vi "Initialize.vi"(8 "error in (no error)":errorcluster, 11 "DSF Buffer Converter Transfers UI in":refnum<class "Default Buffer Converter Transfers UI.lvclass">) -> (0 "error out":errorcluster, 3 "DSF Buffer Converter Transfers UI out":refnum<class "Default Buffer Converter Transfers UI.lvclass">)   [LabVIEW 2019, in "DSF Core.lvlib" / "Default Buffer Converter Transfers UI.lvclass"]
uses:
  Default Buffer Converter Transfers UI.lvclass
  C:/Dev/GitHub/niveristand-data-sharing-framework-custom-device/Core/Classes/User Interface/User Interface.lvclass
  Configurations/Default Buffer Converter Transfer Configuration.lvclass
  C:/Dev/GitHub/niveristand-data-sharing-framework-custom-device/Core/Classes/Configuration/Configuration.lvclass
  Classes/User Interface/User Interface.lvclass
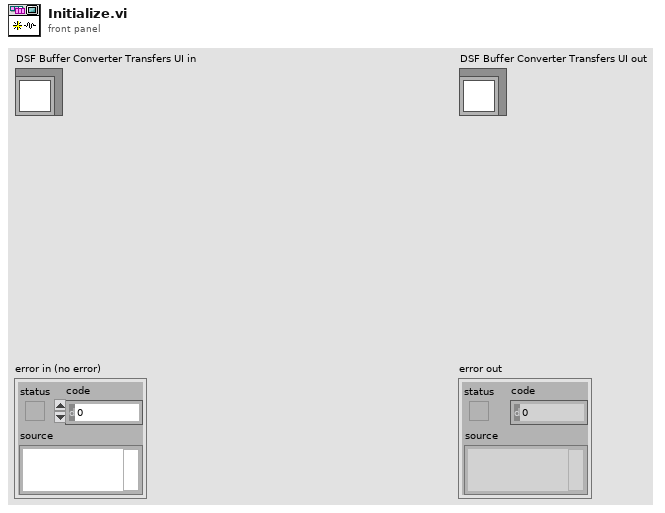
[diagram p1: front panel]
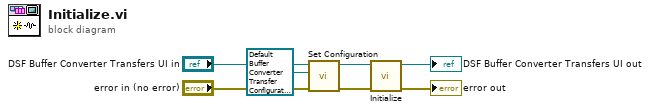
[diagram p0: block diagram]
diagram:
  n1 = call "Set Configuration.vi"("error in (no error)"="error in (no error)", "configuration"=refnum<class "Default Buffer Converter Transfer Configuration.lvclass"> refnum ("DSF Core.lvlib:DSF Buffer Converter Transfer Configuration.lvclass"), "User Interface in"="DSF Buffer Converter Transfers UI in") -> ("error out"=w5:errorcluster, "User Interface out"=w6:refnum<class "Default Buffer Converter Transfers UI.lvclass">)  [unwired: 7 in]
  n2 = call-parent "Initialize.vi"("error in (no error)"=w5, "User Interface in"=w6) -> ("error out"=→"error out":errorcluster, "User Interface out"=→"DSF Buffer Converter Transfers UI out":refnum<class "Default Buffer Converter Transfers UI.lvclass">)  [unwired: 8 in]
